vi "TCP.IP Server for Ripple Detection - Copy.vi"() -> ()   [LabVIEW 2021]
doc: "Demonstrates how to set up a basic TCP connection, send data to the specified port once a connection has been established, and terminate the connection once the data has been sent. This VI is designed to stop if the TCP connection is terminated. The data sent in this example is an array of random numbers."
panel:
  out "Waveform Graph 10":dbl[][](graph)
  in  "loop 1":i32
  in  "loop 2":i32
  in  "Boolean":bool
  in  "Client Closed":string="The client VI closed the connection."
  in  "Stop":bool
  # "Overview: Demonstrates the use of the TCP functions to initialize a TCP server that can send data to a client VI.\nInstructions:\n1. Run the VI.\n2. Open Simple TCP - Client.vi and follow the instructions on its front panel. Note that if you wait longer than 30 seconds to do this after running this VI, it will time out.\n3. Click Stop to stop the VI. Note that if you stop the client VI, this VI will stop automatically."
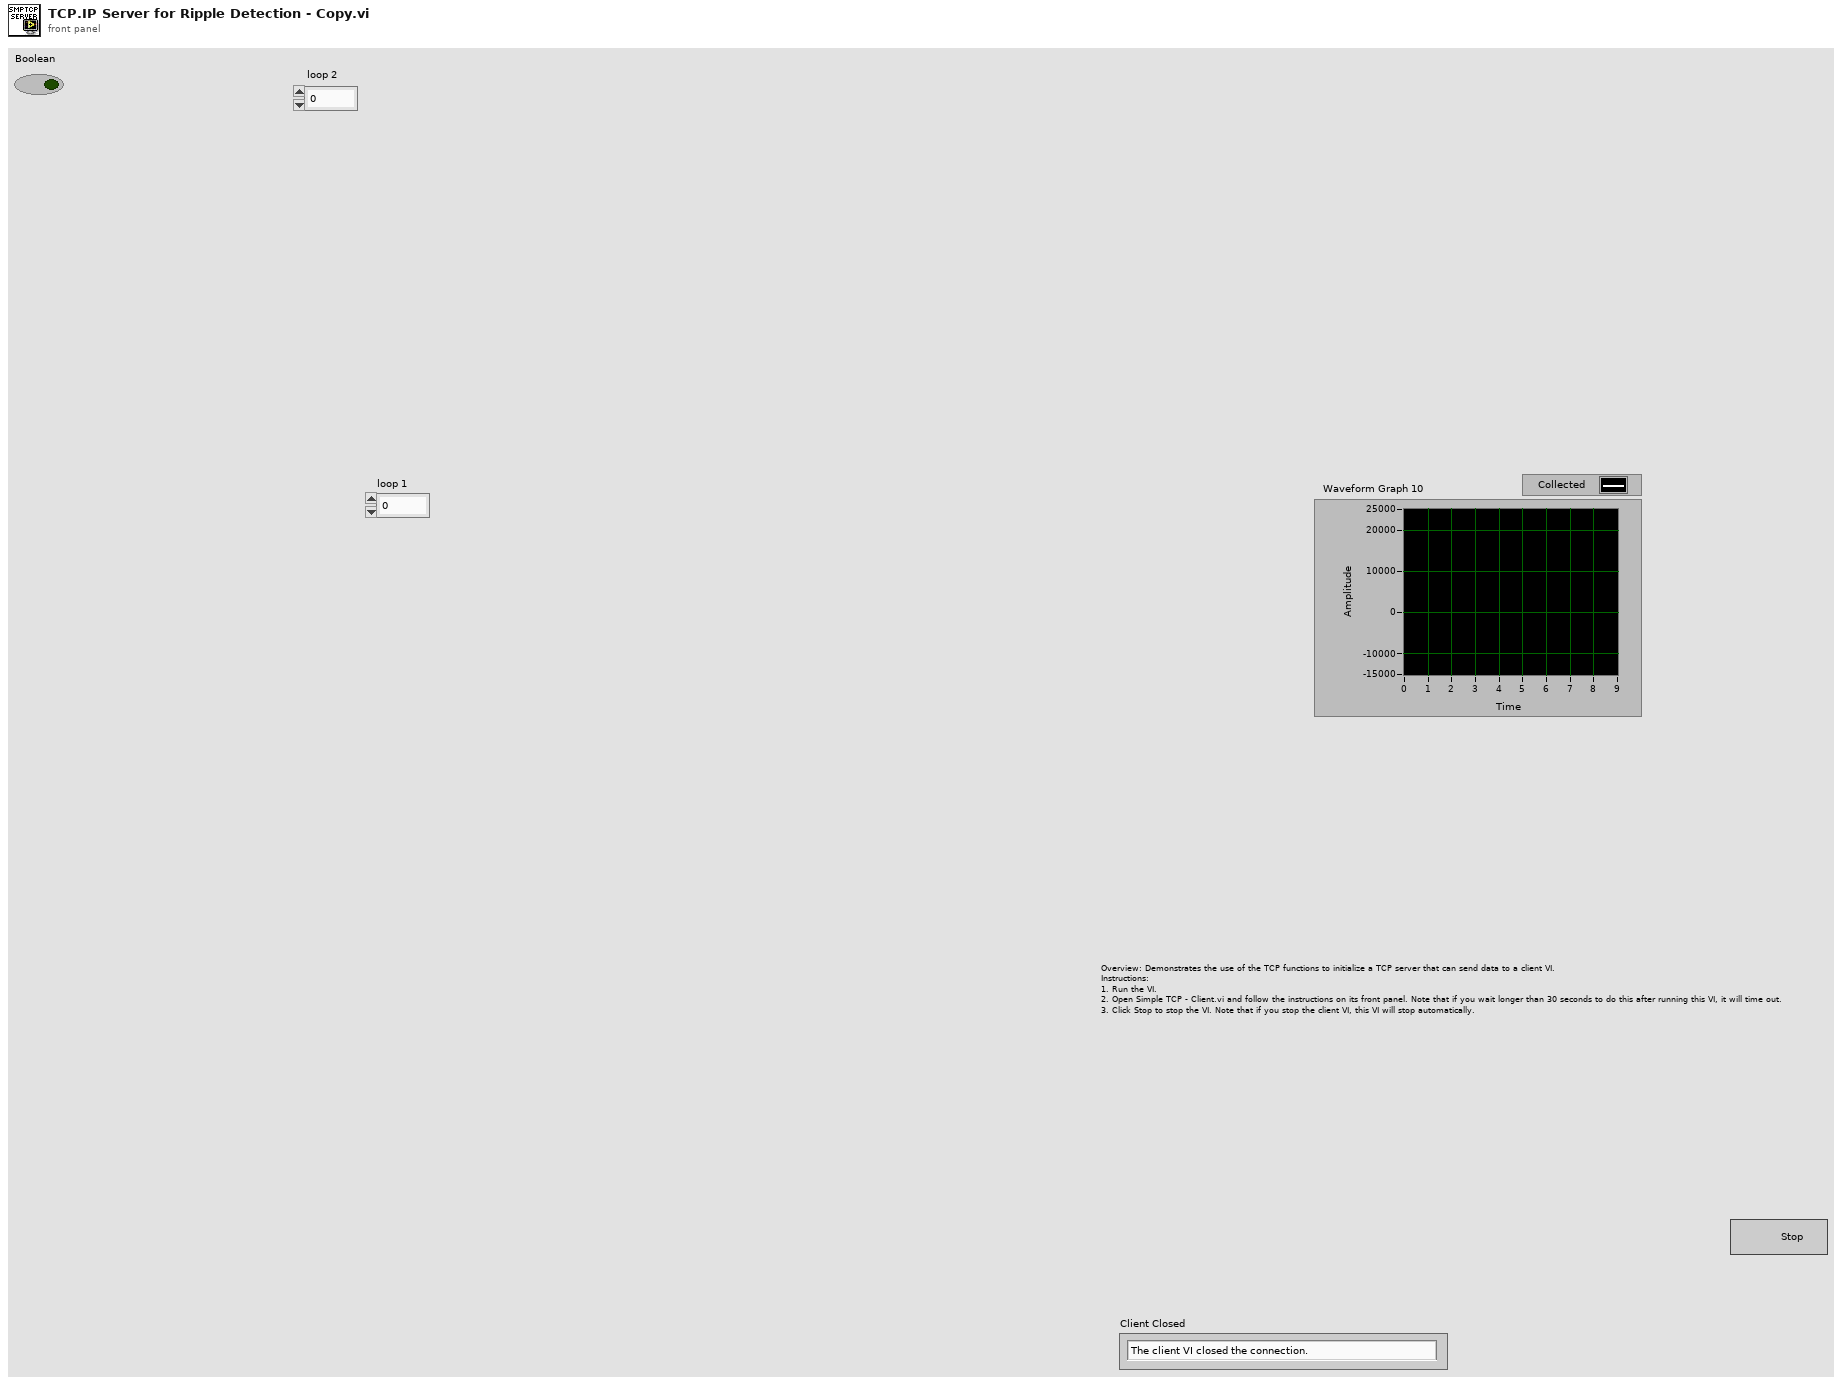
[diagram p1: front panel]
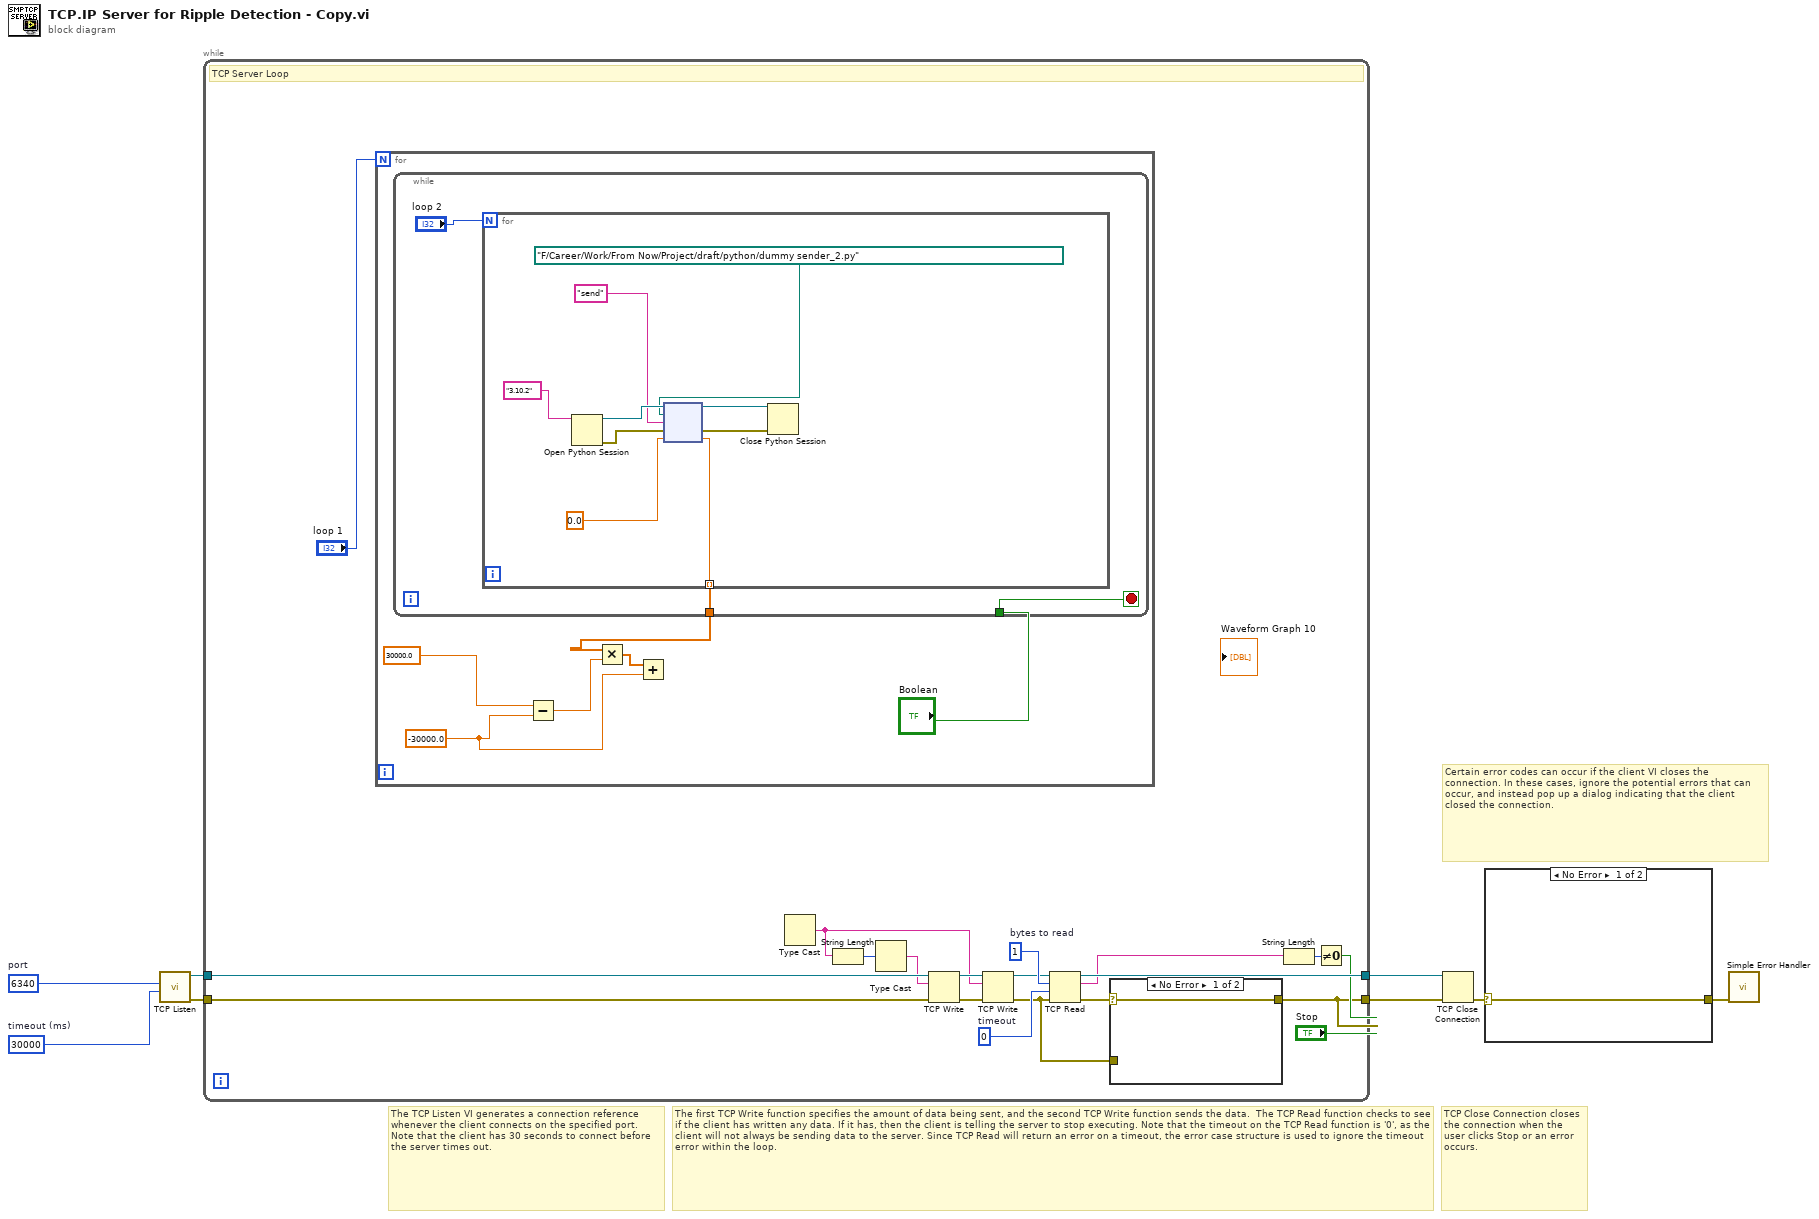
[diagram p0: block diagram]
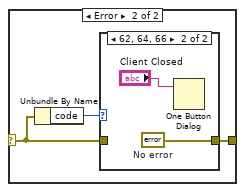
[diagram p2: hidden frame]
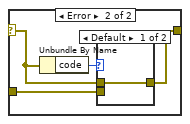
[diagram p4: hidden frame]
diagram:
  w1 = u16 6340  # port
  w2 = 30000  # timeout (ms)
  # "TCP Close Connection closes the connection when the user clicks Stop or an error occurs."
  # "The TCP Listen VI generates a connection reference whenever the client connects on the specified port. Note that the client has 30 seconds to connect before the server times out."
  # "Certain error codes can occur if the client VI closes the connection. In these cases, ignore the potential errors that can occur, and instead pop up a dialog indicating that the client closed the connection."
  # "The first TCP Write function specifies the amount of data being sent, and the second TCP Write function sends the data.  The TCP Read function checks to see if the client has written any data. If it has, then the client is telling the server to stop executing. Note that the timeout on the TCP Read function is '0', as the client will not always be sending data to the server. Since TCP Read will return an error on a timeout, the error case structure is used to ignore the timeout error within the loop."
  n1 = call <vilib>:"TCP Listen.vi"("timeout ms (wait forever: -1)"=w2, "port"=w1) -> ("error out"=w3:errorcluster, "connection ID"=w4:refnum<k5>)  [unwired: 5 in, 3 out]
  n2 = while {
    tunnel: [w11] -> w7
    tunnel: [w17] -> w8
    tunnel: w4 -> [w28]
    tunnel: w3 -> [w21]
    stop <- w22 stop-if-true
    w16 = 0  # timeout
    w19 = 1  # bytes to read
    # "TCP Server Loop"
    n3 = for {
      N: "loop 1" -> [_]
      w31 = -30000.0 ("y")
      n4 = while {
        tunnel: "Boolean" -> [w37]
        tunnel: [w35] -> w29
        stop <- w37 stop-if-true
        n5 = for {
          N: "loop 2" -> [_]
          tunnel: [w38] -> w35 mode=indexing
          n6 = Open Python Session(python version="3.10.2" ("Python version")) -> (session out=w43:refnum<k35>, error out=w46:errorcluster)  [unwired: 2 in]
          n7 = node(w43, path "F:/Career/Work/From Now/Project/draft/python/dummy sender_2.py" ("module path"), "send" ("function name"), w46, 0.0) -> (w44:refnum<k35>, w45:errorcluster, w38:dbl)  [unwired: 2 out]
          n8 = Close Python Session(session in=w44, error in=w45) -> ()  [unwired: 1 out]
        }
      }
      n9 = Subtract(x=30000.0, y=w31) -> (x-y=w34:dbl)
      n10 = Multiply(x=w29, y=w34) -> (x*y=w33:dbl[])
      n11 = Add(x=w33, y=w31) -> ()  [unwired: 1 out]
    }
    n12 = Type Cast() -> (*(type *) &x=w23:string)  [unwired: 1 in, 1 out]
    n13 = String Length(string=w23) -> (length=w25:i32)
    n14 = Type Cast(x=w25) -> (*(type *) &x=w24:string)  [unwired: 1 out]
    n15 = TCP Write(connection ID=w28, data in=w24, error in (no error)=w21) -> (connection ID out=w27:refnum<k5>, error out=w26:errorcluster)  [unwired: 2 out]
    n16 = TCP Write(connection ID=w27, data in=w23, error in (no error)=w26) -> (connection ID out=w18:refnum<k5>, error out=w10:errorcluster)  [unwired: 2 out]
    n17 = TCP Read(connection ID=w18, bytes to read=w19, error in (no error)=w10, 9:w16) -> (connection ID out=w17:refnum<k5>, data out=w14:string, error out=w12:errorcluster)  [unwired: 1 out]
    n18 = case shown="No Error" w12 {
      selector: w12 -> [w47 w50]
      tunnel: [w47 w48] -> w11
      tunnel: w10 -> [_ w49]
      frame No Error {
      }
      frame Error {
        n19 = Unbundle By Name(w50) -> ("code"=w51:i32)
        n20 = case shown="Default" w51 {
          tunnel: w50 -> [w52 _]
          tunnel: w49 -> [_ w53]
          tunnel: [w52 w53] -> w48
          frame Default {
          }
          frame 56 {
          }
        }
      }
    }
    n21 = String Length(string=w14) -> (length=w15:i32)
    n22 = Not Equal To 0?(x=w15) -> (x != 0?=w13:bool)
    n23 = Compound Arithmetic op=OR(w13, w11, "Stop") -> (w22:bool)
  }
  n24 = TCP Close Connection(connection ID=w8, error in (no error)=w7) -> (error out=w6:errorcluster)  [unwired: 2 out]
  n25 = case shown="No Error" w6 {
    selector: w6 -> [w54 w56]
    tunnel: [w54 w55] -> w5
    frame No Error {
    }
    frame Error {
      n26 = Unbundle By Name(w56) -> ("code"=w57:i32)
      n27 = case shown="62, 64, 66" w57 {
        tunnel: w56 -> [w58 _]
        tunnel: [w58 w60] -> w55
        frame Default {
        }
        frame 62, 64, 66 {
          w60 = errorcluster {"status"=FALSE, "code"=0, "source"=""}  # No error
          n28 = One Button Dialog(message="Client Closed") -> ()  [unwired: 1 in, 1 out]
        }
      }
    }
  }
  n29 = call <vilib>:"Simple Error Handler.vi"("error in (no error)"=w5) -> ()  [unwired: 1 in, 8 out]
